vi "get_roi_intensity.vi"(8 "Error In":errorcluster, 10 "ROI In":T2, 11 "Image":T1) -> (0 "Error Out":errorcluster, 3 "Intensity":dbl)   [LabVIEW 2019]
uses:
  <vilib>/vision/Image Controls.llb/IMAQ Image.ctl
  <vilib>/vision/NI_Vision_Development_Module.lvlib
panel:
  out "Image 2":T1(plugin-control)
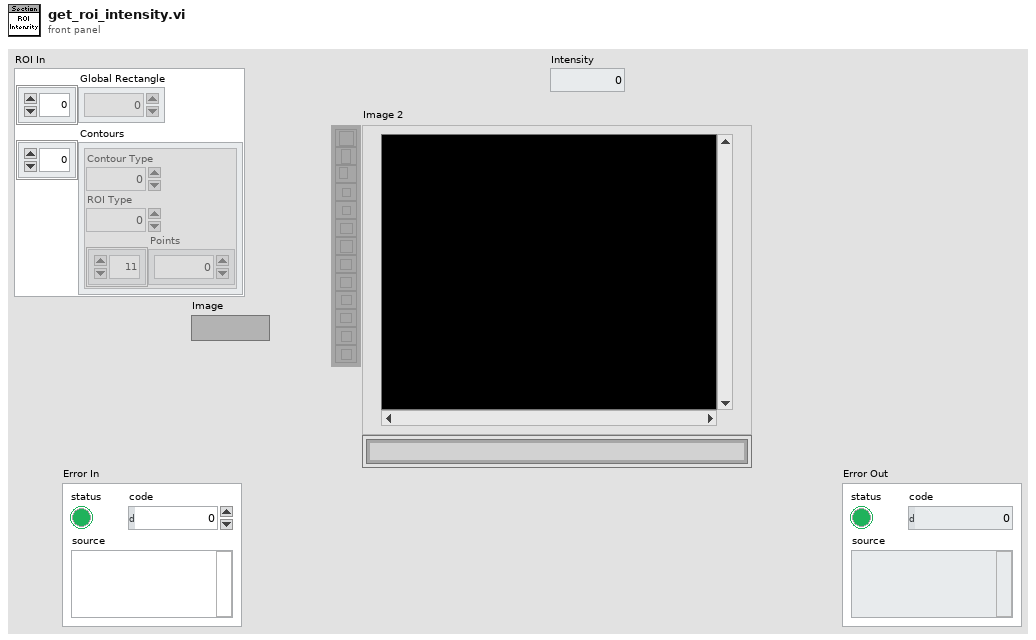
[diagram p1: front panel]
types:
  T1 = typedef "IMAQ Image.ctl" = refnum<image>
  T2 = cluster{"Global Rectangle":i32[], "Contours":cluster{"Contour Type":u32, "ROI Type":u32, "Points":i32[]}[]}
  T3 = cluster{"Mean Value":sgl, "Standard Variation":sgl, "Minimal Value":sgl, "Maximal Value":sgl, "Area (calibrated)":sgl, "Area (pixels)":u32, "%":sgl, "Calibration Valid":bool}
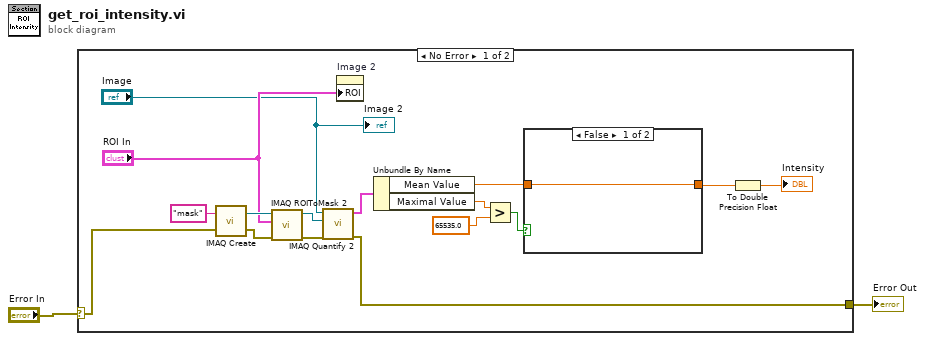
[diagram p0: block diagram]
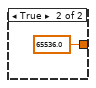
[diagram p2: hidden frame]
diagram:
  n1 = case shown="No Error" "Error In" {
    selector: "Error In" -> [w8 w21]
    tunnel: [w7 w21] -> w1
    frame No Error {
      n2 = call "IMAQ Create"("Image Name"="mask", "error in (no error)"=w8) -> ("New Image"=w15:T1, "error out"=w14:errorcluster)  [unwired: 3 in]
      n3 = call "IMAQ ROIToMask 2"("error in (no error)"=w14, "ROI Descriptor"="ROI In", "Image"=w15) -> ("error out"=w18:errorcluster, "Image Out"=w17:T1)  [unwired: 6 in, 1 out]
      n4 = call "IMAQ Quantify 2"("error in (no error)"=w18, "Image Mask"=w17, "Image"="Image") -> ("error out"=w7:errorcluster, "Global Report"=w13:T3)  [unwired: 6 in, 1 out]
      n5 = property on="Image 2" class="ImageControl"("ROI"="ROI In") -> ()  [unwired: 2 in, 2 out]
      n6 = Unbundle By Name(w13) -> ("Mean Value"=w9:sgl, "Maximal Value"=w11:sgl)
      n7 = Greater?(x=w11, y=sgl 65535.0) -> (0:w12:bool)
      n8 = case shown="False" w12 {
        tunnel: w9 -> [w19 _]
        tunnel: [w19 sgl 65536.0 ("Mean Value")] -> w5
        frame False {
        }
        frame True {
        }
      }
      n9 = To Double Precision Float(number=w5) -> (double precision float=→"Intensity":dbl)
      "Image 2" <- "Image"
    }
    frame Error {
    }
  }
  "Error Out" <- w1
